vi "Convert Data to Waveforms.vi"   [LabVIEW 2014, in "NI_EP_Power Quality.lvlib"]
doc: "Converts resampled voltage and current data to voltage and current waveforms of different line configurations. This VI also arranges the order of the elements in the waveforms of each three-phase electrical power system for further measurement. For example, the orders are A-B-C-N for the four-channel method and A-B-C for the three-channel method. You must manually select the polymorphic instance you want to use."
uses:
  <vilib>/addons/Electrical Power/PQ/NI_EP_Power Quality.lvlib
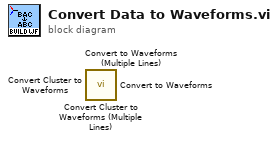
[diagram p0: block diagram]
diagram:
  n1 = call <vilib>:"Convert Cluster to Waveforms (Multiple Lines).vi"() -> ()  [unwired: 11 in, 5 out]
  n2 = call <vilib>:"Convert to Waveforms (Multiple Lines).vi"() -> ()  [unwired: 11 in, 5 out]
  n3 = call <vilib>:"Convert Cluster to Waveforms.vi"() -> ()  [unwired: 11 in, 5 out]
  n4 = call <vilib>:"Convert to Waveforms.vi"() -> ()  [unwired: 11 in, 5 out]
